vi "GetVerticalChannelDataFromSettings.vi"(8 "error in (no error)":errorcluster, 11 "TektronixDPO in":refnum<class "TektronixDPO.lvclass">) -> (0 "error out":errorcluster, 3 "TektronixDPO Out":refnum<class "TektronixDPO.lvclass">)   [LabVIEW 2013, in "TektronixDPO.lvclass"]
doc: "Retreive the vertical parameters relative to the specified channel from the Settings Cluster and write them into a TektronixDPO_PhysicalDevice object"
uses:
  TektronixDPO.lvclass
  shared/Typdefs/Choice78.ctl
  shared/Typdefs/Choice79.ctl
  shared/Typdefs/Choice11.ctl
  shared/OnOffTypeDef.ctl
  shared/Typdefs/Choice80.ctl
  TektronixDPO.lvclass/TektronixDPO.ctl
  SupportClasses/TektronixDPOPhysicalDevice/TektronixDPO_PhysicalDevice.lvclass
  shared/UtilsLib/ClusterManipulation/GetClusterElementByName(Variant).vi
  shared/UtilsLib/ClusterManipulation/GetClusterElementByName.lvlib
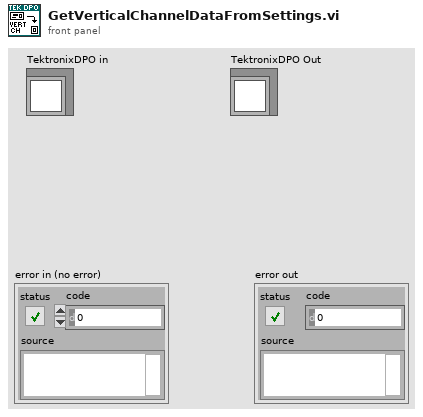
[diagram p1: front panel]
types:
  T1 = typedef "Choice80.ctl" = u16
  T2 = typedef "OnOffTypeDef.ctl" = enum16{"off", "on"}
  T3 = typedef "Choice11.ctl" = enum16{"AC", "DC", "Ground"}
  T4 = typedef "Choice79.ctl" = enum16{"FULL", "250 MHz", "150 MHz", "20 MHz"}
  T5 = typedef "Choice78.ctl" = enum16{"1M", "75", "50"}
  T6 = typedef "settings_TypDef.ctl" = cluster{"resourcename":string, "timeout":T7, "LocalSavingPath":path, "Save":T2, "Names":cluster{"Channel0":string, "Channel1":string, "Channel2":string, "Channel3":string, "Channel4":string}, "Calculations":T8, "NumChannels":T7, "NumMeasurements":T7, "NumPoints":T7, "waveformattributes":string, "Measurements":cluster{"Channel0":T7, "Channel1":T7, "Channel2":T7, "Channel3":T7}, "EnableMeasurements":T2, "Trigger":T14, "EnableReadWaveformInfo":T2, "probeattenuation":cluster{"Channel0":T7, "Channel1":T7, "Channel2":T7, "Channel3":T7}, "offset":cluster{"Channel0":T7, "Channel1":T7, "Channel2":T7, "Channel3":T7}, "Horizontal":T19, "verticalrange":cluster{"Channel0":T7, "Channel1":T7, "Channel2":T7, "Channel3":T7}, "Impedance":cluster{"Channel0":T5, "Channel1":T5, "Channel2":T5, "Channel3":T5}, "channelenabled":cluster{"Channel0":T2, "Channel1":T2, "Channel2":T2, "Channel3":T2}, "bandwidth":cluster{"Channel0":T4, "Channel1":T4, "Channel2":T4, "Channel3":T4}, "coupling":cluster{"Channel0":T3, "Channel1":T3, "Channel2":T3, "Channel3":T3}}
  T7 = typedef "BaseDriver.lvclass/numericVariable_TypeDef.ctl" = cluster{"Value":dbl, "Min":dbl, "Max":dbl, "StepSize":dbl, "Tolerance":dbl, "ValueActual":dbl}
  T8 = typedef "analysisTypDEf.ctl" = cluster{"Additional":T9, "Linked":T10, "Method":T12}
  T9 = typedef "additionalAnalysisCluster_TypDef.ctl" = cluster{"Analysis1":dbl, "Analysis2":dbl, "Analysis3":dbl, "Analysis4":dbl, "Analysis5":dbl, "Analysis6":dbl, "Analysis7":dbl, "Analysis8":dbl, "Analysis9":dbl, "Analysis10":dbl}
  T10 = typedef "LinkedChannelsCluster_TypDef.ctl" = cluster{"Analysis1":T11, "Analysis2":T11, "Analysis3":T11, "Analysis4":T11, "Analysis5":T11, "Analysis6":T11, "Analysis7":T11, "Analysis8":T11, "Analysis9":T11, "Analysis10":T11}
  T11 = typedef "channels_TypDef.ctl" = enum16{"Channel0", "Channel1", "Channel2", "Channel3", "Channel4", "Channel5", "Channel6", "Channel7", "n/a"}
  T12 = typedef "methodCluster_TypDEf.ctl" = cluster{"Analysis1":T13, "Analysis2":T13, "Analysis3":T13, "Analysis4":T13, "Analysis5":T13, "Analysis6":T13, "Analysis7":T13, "Analysis8":T13, "Analysis9":T13, "Analysis10":T13}
  T13 = typedef "method_TypDef.ctl" = enum16{"n/a", "max", "min", "energy", "trigger", "maxtime", "mintime"}
  T14 = typedef "TriggerCluster.ctl" = cluster{"Mode":T15, "Source":T16, "Coupling":T17, "Slope":T18, "Low Level":dbl}
  T15 = typedef "Choice73.ctl" = enum16{"Immediate", "Analog Edge"}
  T16 = typedef "Choice74.ctl" = enum16{"Channel 1", "Channel 2", "Channel 3", "Channel 4", "AC Line", "Aux", "Digital Channel 0", "Digital Channel 1", "Digital Channel 2", "Digital Channel 3", "Digital Channel 4", "Digital Channel 5", "Digital Channel 6", "Digital Channel 7", "Digital Channel 8", "Digital Channel 9", "Digital Channel 10", "Digital Channel 11", "Digital Channel 12", "Digital Channel 13", "Digital Channel 14", "Digital Channel 15", "RF"}
  T17 = typedef "Choice75.ctl" = enum16{"DC", "HF Reject", "LF Reject", "Noise Reject", "AC"}
  T18 = typedef "Choice76.ctl" = enum16{"Rising", "Falling"}
  T19 = typedef "Horizontal.ctl" = cluster{"time_window":dbl, "resolution":T20}
  T20 = typedef "Choice77.ctl" = enum16{"1E+3", "10E+3", "100E+3", "1E+6", "5E+6", "10E+6"}
  T21 = typedef "Choice78.ctl" = u16
  T22 = cluster{"Channel":T21, "offset":dbl, "verticalrange":dbl, "Impedance":u16, "Probe Attenuation":dbl, "Vertical Coupling":u16, "Bandwidth":u16, "Enabled":bool}
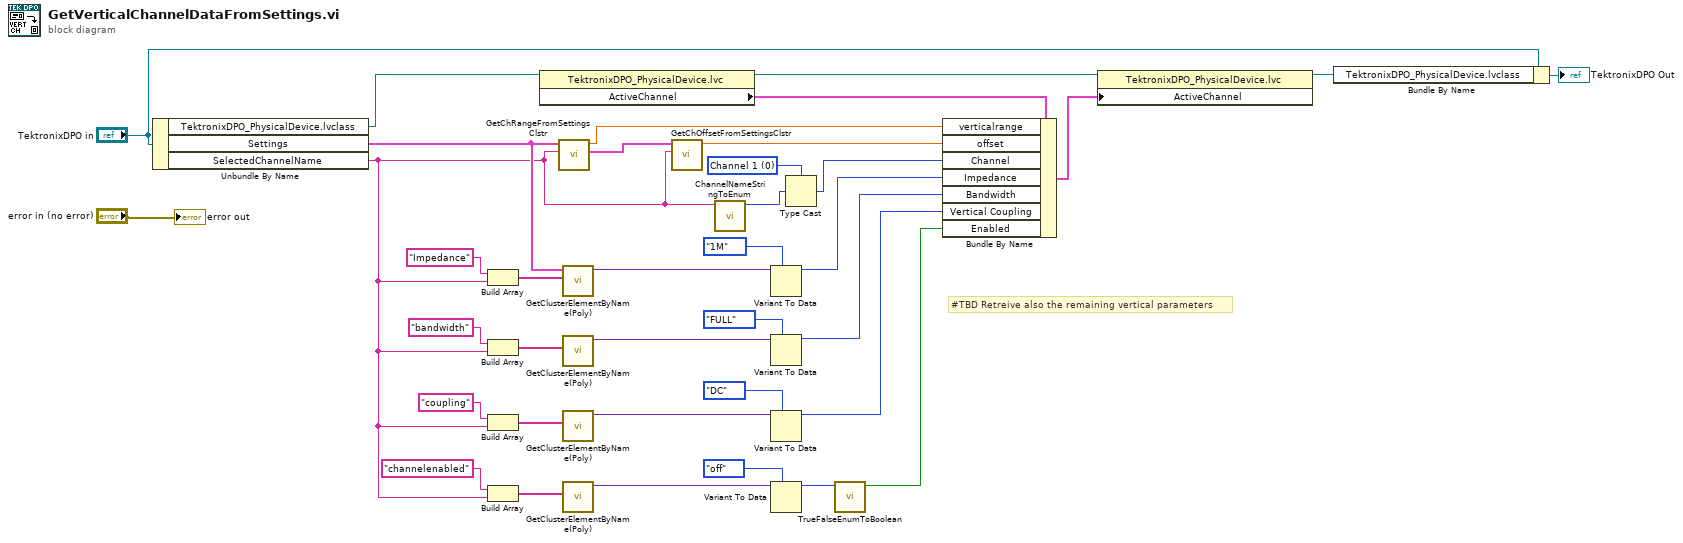
[diagram p0: block diagram]
diagram:
  w3 = T1 0 items=["Channel 1", "Channel 2", "Channel 3", "Channel 4", "Math", "Reference 1", "Reference 2", "Reference 3", "Reference 4", "Bus 1", "Bus 2"] ("ActiveChannel.Channel")
  # "#TBD Retreive also the remaining vertical parameters"
  n1 = Unbundle By Name("TektronixDPO in") -> ("TektronixDPO_PhysicalDevice.lvclass"=w34:refnum<class "TektronixDPO_PhysicalDevice.lvclass">, "Settings"=w16:T6, "SelectedChannelName"=w7:string)
  n2 = Build Array("Impedance" ("string"), w7) -> (w25:string[])
  n3 = Build Array("bandwidth" ("string"), w7) -> (w20:string[])
  n4 = Build Array("coupling" ("string"), w7) -> (w19:string[])
  n5 = Build Array("channelenabled" ("string"), w7) -> (w8:string[])
  n6 = property class="TektronixDPO_PhysicalDevice.lvc"(reference=w34) -> (reference out=w33:refnum<class "TektronixDPO_PhysicalDevice.lvclass">, "ActiveChannel"=w37:T22)  [unwired: 1 in, 1 out]
  n7 = call "GetChRangeFromSettingsClstr.vi"("ChannelName"=w7, "Settings"=w16) -> ("SettingsOut"=w28:T6, "ValueOut"=w36:dbl)  [unwired: 8 in]
  n8 = call-poly "GetClusterElementByName(Poly).vi"("ElementHierarchy"=w25, "Cluster"=w16) -> ("Element"=w23:variant)  [unwired: 8 in, 1 out]
  n9 = call-poly "GetClusterElementByName(Poly).vi"("ElementHierarchy"=w20) -> ("Element"=w15:variant)  [unwired: 9 in, 1 out]
  n10 = call-poly "GetClusterElementByName(Poly).vi"("ElementHierarchy"=w19) -> ("Element"=w17:variant)  [unwired: 9 in, 1 out]
  n11 = call-poly "GetClusterElementByName(Poly).vi"("ElementHierarchy"=w8) -> ("Element"=w10:variant)  [unwired: 9 in, 1 out]
  n12 = call "GetChOffsetFromSettingsClstr.vi"("ChannelName"=w7, "Settings"=w28) -> ("ValueOut"=w35:dbl)  [unwired: 9 in]
  n13 = call "ChannelNameStringToEnum.vi"("ChannelName"=w7) -> ("Channel (0: Channel 1)"=w1:T1)  [unwired: 10 in]
  n14 = Variant To Data(type=Choice78."1M" ("Impedance"), Variant=w23) -> (data=w22:T5)  [unwired: 1 in, 1 out]
  n15 = Variant To Data(type=Choice79."FULL" ("Channel0"), Variant=w15) -> (data=w13:T4)  [unwired: 1 in, 1 out]
  n16 = Variant To Data(type=Choice11."DC" ("Channel0"), Variant=w17) -> (data=w12:T3)  [unwired: 1 in, 1 out]
  n17 = Variant To Data(type=OnOffTypeDef."off" ("Channel0"), Variant=w10) -> (data=w5:T2)  [unwired: 1 in, 1 out]
  n18 = Type Cast(type=w3, x=w1) -> (*(type *) &x=w2:T1)
  n19 = call "TrueFalseEnumToBoolean.vi"("ChannelOn"=w5) -> ("selection"=w4:bool)  [unwired: 9 in, 1 out]
  n20 = Bundle By Name(cluster=w37, "verticalrange"=w36, "offset"=w35, "Channel"=w2, "Impedance"=w22, "Bandwidth"=w13, "Vertical Coupling"=w12, "Enabled"=w4) -> (w32:T22)
  n21 = property class="TektronixDPO_PhysicalDevice.lvc"(reference=w33, "ActiveChannel"=w32) -> (reference out=w30:refnum<class "TektronixDPO_PhysicalDevice.lvclass">)  [unwired: 1 in, 1 out]
  n22 = Bundle By Name(cluster="TektronixDPO in", "TektronixDPO_PhysicalDevice.lvclass"=w30) -> (→"TektronixDPO Out":refnum<class "TektronixDPO.lvclass">)
  "error out" <- "error in (no error)"
